vi "Error_Format.vi"(0 "FIFO IN":T1(array[cluster]), 2 "Error Code IN":u32, 3 "Warning Code IN":u32, 4 "Error Bit":u32, 5 "Warning Bit":u32, 8 "Source":string, 9 "Comment":string) -> (14 "FIFO OUT":T1(array[cluster]), 16 "Error Code OUT":u32, 17 "Warning Code OUT":u32)   [LabVIEW 2019]
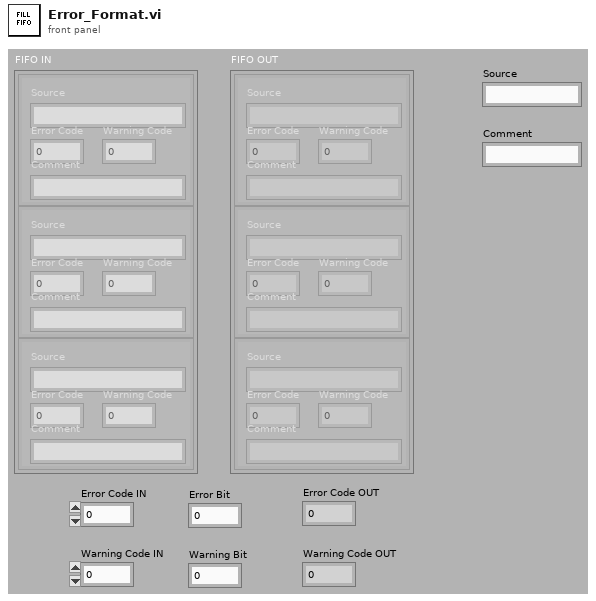
[diagram p1: front panel]
types:
  T1 = cluster{"Source":string, "Error Code":u32, "Warning Code":u32, "Comment":string}[]
  T2 = cluster{"Source":string, u32, u32, "Comment":string}
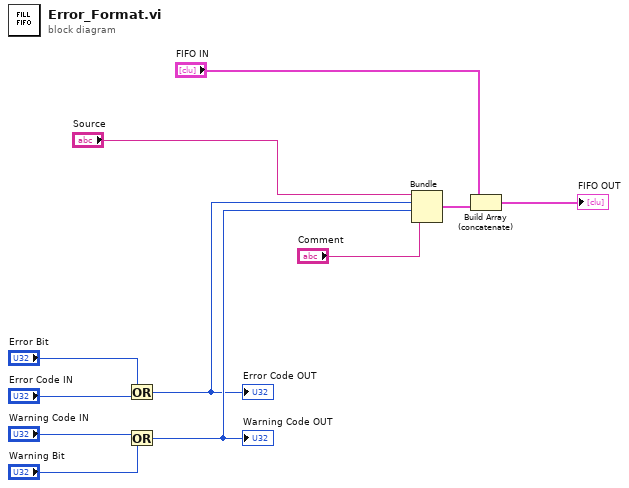
[diagram p0: block diagram]
diagram:
  n1 = Or(x="Error Bit", y="Error Code IN") -> (x .or. y?=w4:u32)
  "Error Code OUT" <- w4
  n2 = Or(x="Warning Code IN", y="Warning Bit") -> (x .or. y?=w5:u32)
  "Warning Code OUT" <- w5
  n3 = Bundle("Source"="Source", w4, w5, "Comment"="Comment") -> (w11:T2)  [unwired: 1 in]
  n4 = Build Array (concatenate)("FIFO IN", w11) -> (→"FIFO OUT":T1)
